vi "CCDumpWorklist.vi"(8 "error in (no error)":errorcluster, 9 "patientID":string="C:\\Users\\Simon\\Dropbox\\Medimatic\\ProjectVerLV2011\\tmp.dcm", 10 "index":i32, 11 "Find":refnum<k24>) -> (0 "error out":errorcluster)   [LabVIEW 2013, in "main.lvlib" / "ClearCanvasLibrary.lvlib"]
uses:
  ClearCanvasLibrary.lvlib
  C:/Users/Simon/SkyDrive/LabView/2013/DM2020/DICOM/ClearCanvasNewBuild/ClearCanvas.Dicom.dll
  ClearCanvasNewBuild/ClearCanvas.Dicom.dll
  Globals/DataPathGlobalVariable.vi
  main.lvlib
  <userlib>/_OpenG.lib/file/file.llb/File Exists - Scalar__ogtk.vi
panel:
  out "Dump":string
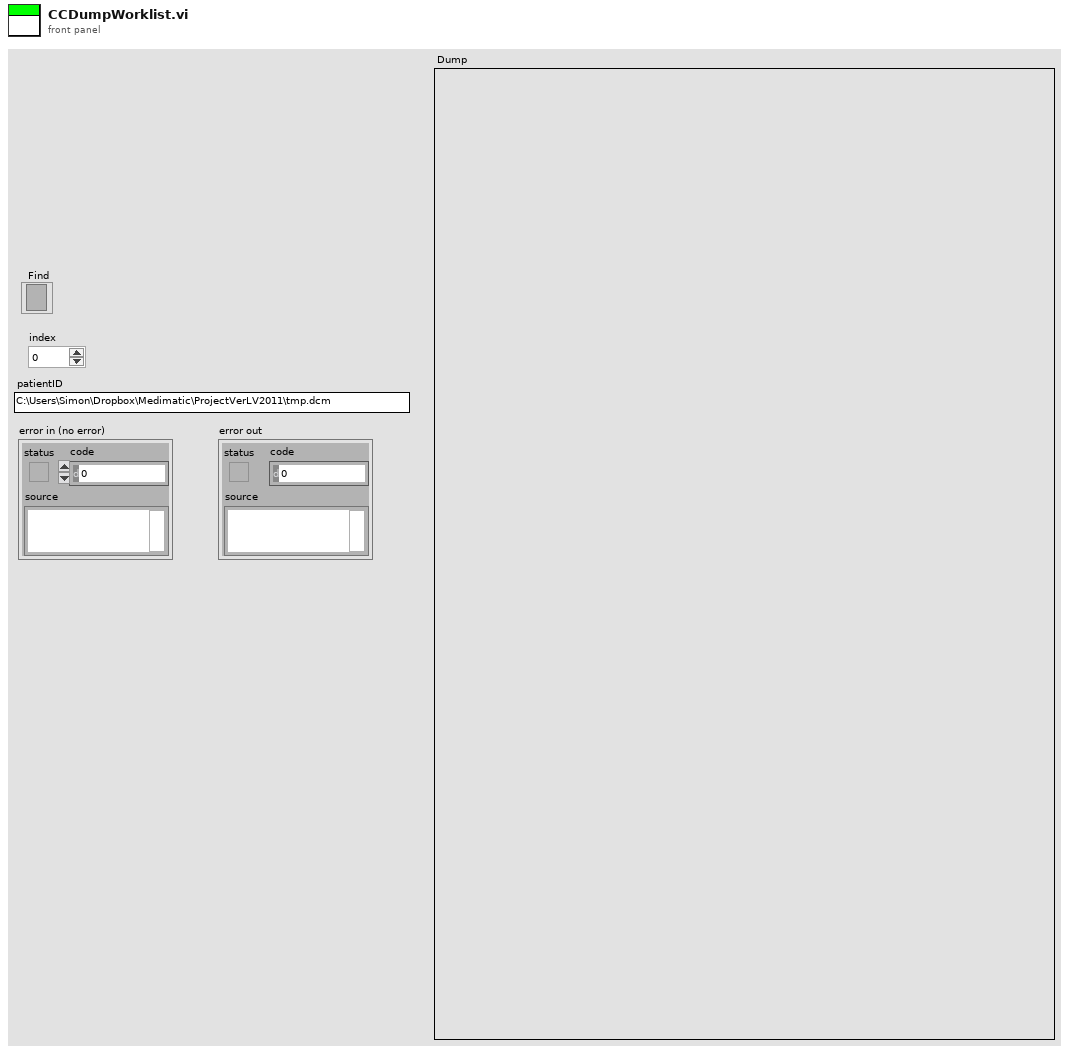
[diagram p1: front panel]
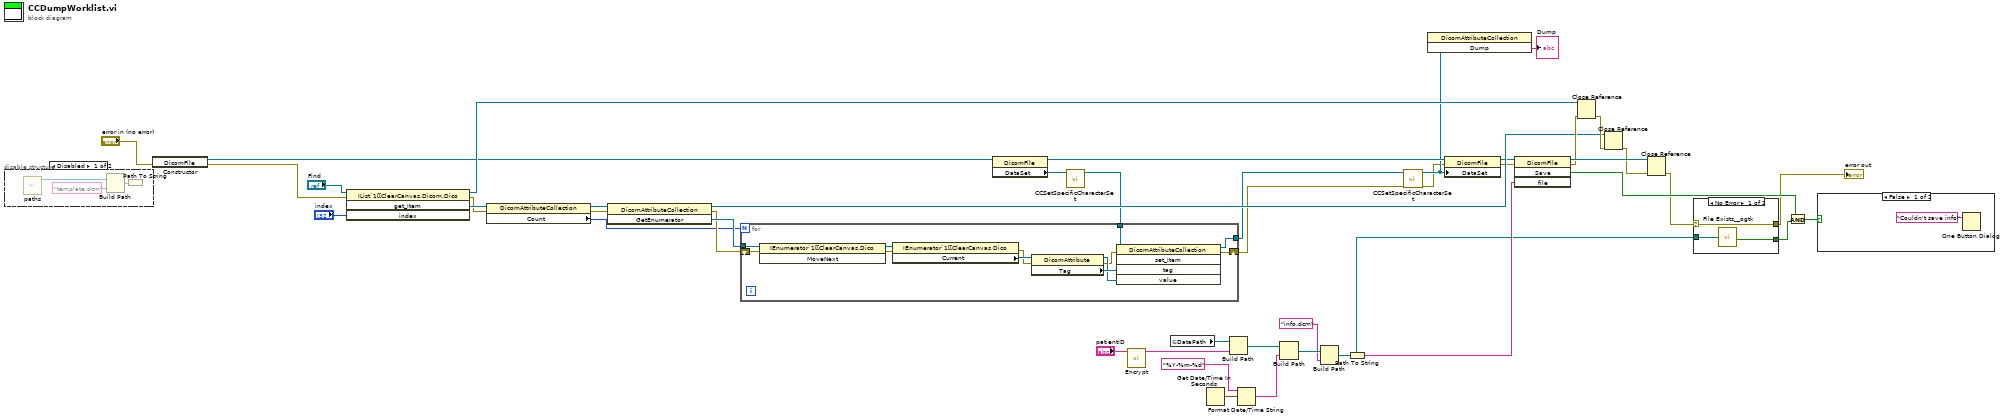
[diagram p0: block diagram]
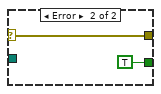
[diagram p3: hidden frame]
diagram:
  n1 = disable-structure shown="Disabled" {
    frame Disabled {
      n2 = call "paths.vi"() -> ("PubAppData"=w46:path)  [unwired: 8 in, 3 out]
      n3 = Build Path(base path=w46, name or relative path="template.dcm") -> (appended path=w45:path)
      n4 = Path To String(path=w45) -> ()  [unwired: 1 out]
    }
    frame Enabled {
    }
  }
  n5 = constructor class="DicomFile"(error in="error in (no error)") -> (reference out=w2:refnum<k24>, error out=w1:errorcluster)  [unwired: 2 in, 1 out]
  n6 = invoke class="IList`1[[ClearCanvas.Dicom.Dico" method="get_Item"(reference="Find", error in=w1, "index"="index") -> (reference out=w21:refnum<k24>, error out=w19:errorcluster, "get_Item"=w20:refnum<k24>)  [unwired: 1 in, 1 out]
  n7 = property class="DicomAttributeCollection"(reference=w20, error in=w19) -> (reference out=w18:refnum<k24>, error out=w17:errorcluster, "Count"=w14:i32)
  n8 = invoke class="DicomAttributeCollection" method="GetEnumerator"(reference=w18, error in=w17) -> (reference out=w22:refnum<k24>, error out=w15:errorcluster, "GetEnumerator"=w16:refnum<k24>)  [unwired: 1 in]
  n9 = property class="DicomFile"(reference=w2) -> (reference out=w12:refnum<k24>, "DataSet"=w4:refnum<k24>)  [unwired: 1 in, 1 out]
  n10 = call "CCSetSpecificCharacterSet.vi"(".NET Refnum in"=w4) -> (".NET Refnum out"=w3:refnum<k24>)  [unwired: 9 in, 1 out]
  n11 = for {
    N: w14 -> [_]
    tunnel: w3 -> [w59]
    tunnel: w16 -> [w58]
    shift-right: [w52] -> w7
    shift-left: w15 -> [w49]
    tunnel: [w48] -> w8
    n12 = invoke class="IEnumerator`1[[ClearCanvas.Dico" method="MoveNext"(reference=w58, error in=w49) -> (reference out=w57:refnum<k24>, error out=w55:errorcluster)  [unwired: 1 in, 1 out]
    n13 = property class="IEnumerator`1[[ClearCanvas.Dico"(reference=w57, error in=w55) -> (error out=w51:errorcluster, "Current"=w56:refnum<k24>)  [unwired: 1 out]
    n14 = property class="DicomAttribute"(reference=w56, error in=w51) -> (reference out=w53:refnum<k24>, error out=w50:errorcluster, "Tag"=w54:refnum<k24>)
    n15 = invoke class="DicomAttributeCollection" method="set_Item"(reference=w59, error in=w50, "tag"=w54, "value"=w53) -> (reference out=w48:refnum<k24>, error out=w52:errorcluster)  [unwired: 1 in, 3 out]
  }
  n16 = call "Encrypt.vi"("Input"="patientID") -> ("Output"=w30:string)  [unwired: 10 in]
  n17 = global read "DataPathGlobalVariable.vi" "DataPath"() -> (w38:path)
  n18 = Get Date/Time In Seconds() -> (seconds since 1Jan1904=w37:timestamp)
  n19 = Build Path(base path=w38, name or relative path=w30) -> (appended path=w35:path)
  n20 = Format Date/Time String(time format string (%c)="%Y-%m-%d", seconds (now)=w37) -> (date/time string=w34:string)  [unwired: 1 in]
  n21 = Build Path(base path=w35, name or relative path=w34) -> (appended path=w33:path)
  n22 = Build Path(base path=w33, name or relative path="info.dcm") -> (appended path=w10:path)
  n23 = Path To String(path=w10) -> (string=w23:string)
  n24 = call "CCSetSpecificCharacterSet.vi"("error in (no error)"=w7, ".NET Refnum in"=w8) -> ("error out"=w5:errorcluster, ".NET Refnum out"=w6:refnum<k24>)  [unwired: 8 in]
  n25 = invoke class="DicomAttributeCollection" method="Dump"(reference=w6) -> ("Dump"=→"Dump":string)  [unwired: 2 in, 2 out]
  n26 = property class="DicomFile"(reference=w12, error in=w5, "DataSet"=w6) -> (reference out=w13:refnum<k24>, error out=w11:errorcluster)
  n27 = invoke class="DicomFile" method="Save"(reference=w13, error in=w11, "file"=w23) -> (reference out=w44:refnum<k24>, error out=w40:errorcluster, "Save"=w26:bool)  [unwired: 1 in, 1 out]
  n28 = Close Reference(reference=w21, error in (no error)=w40) -> (error out=w41:errorcluster)
  n29 = Close Reference(reference=w22, error in (no error)=w41) -> (error out=w39:errorcluster)
  n30 = Close Reference(reference=w44, error in (no error)=w39) -> (error out=w25:errorcluster)
  n31 = case shown="No Error" w25 {
    selector: w25 -> [w61 w64]
    tunnel: [w62 TRUE ("exists")] -> w27
    tunnel: [w61 w64] -> w24
    tunnel: w10 -> [w60 _]
    frame No Error {
      n32 = call-poly <userlib>:"File Exists__ogtk.vi"("file path"=w60) -> ("exists"=w62:bool)  [unwired: 6 in, 1 out]
    }
    frame Error {
    }
  }
  "error out" <- w24
  n33 = And(x=w26, y=w27) -> (x .and. y?=w28:bool)
  n34 = case shown="False" w28 {
    frame False {
      n35 = One Button Dialog(message="Couldn't save info") -> ()  [unwired: 1 in, 1 out]
    }
    frame True {
    }
  }
